vi "Update Any Values to UI.vi"(0 "Measurement Client Wrapper":refnum<class "Measurement Client Wrapper.lvclass">, 11 "error in":errorcluster) -> (4 "Measurement Client Wrapper out":refnum<class "Measurement Client Wrapper.lvclass">, 15 "error out":errorcluster)   [LabVIEW 2020, in "Measurement Client Wrapper.lvclass"]
uses:
  Measurement Client Wrapper.lvclass
  Measurement Client Wrapper.lvclass/Measurement Client Wrapper.ctl
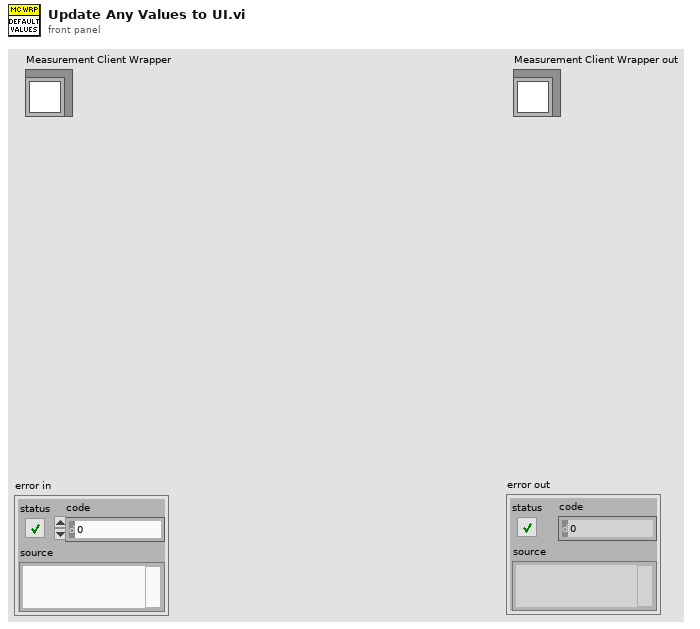
[diagram p1: front panel]
types:
  T1 = typedef "Measurement Client Wrapper.lvclass/MeasurementConfigurationParameters.ctl" = cluster{"protobuf_id":u32, "type":T2, "name":string, "repeated":bool}
  T2 = typedef "Measurement_client-release.lvlib/ni_measurements_v1_Type.ctl" = enum32{"TYPE_UNSPECIFIED", "TYPE_DOUBLE", "TYPE_FLOAT", "TYPE_INT64", "TYPE_UINT64", "TYPE_INT32", "TYPE_FIXED64", "TYPE_FIXED32", "TYPE_BOOL", "TYPE_STRING", "TYPE_GROUP", "TYPE_MESSAGE", "TYPE_BYTES", "TYPE_UINT32", "TYPE_ENUM", "TYPE_SFIXED32", "TYPE_SFIXED64", "TYPE_SINT32", "TYPE_SINT64"}
  T3 = typedef "Measurement Client Wrapper.lvclass/Control UI MetaData.ctl" = cluster{"Name":string, "Parent":string, "LabVIEW DataType":T4, "Measurement DataType":T2, "Value":variant, "1D Array?":bool}
  T4 = typedef "NI_Data Type.lvlib/Data Type.ctl" = enum8{"Invalid Type", "Void", "I8", "I16", "I32", "I64", "U8", "U16", "U32", "U64", "Single Float", "Double Float", "Extended Float", "Single Complex", "Double Complex", "Extended Complex", "Enum U8", "Enum U16", "Enum U32", "Enum U64", "Single Float With Unit", "Double Float With Unit", "Extended Float With Unit", "Single Complex with Unit", "Double Complex with Unit", "Extended Complex with Unit", "Boolean", "String", "Path", "Picture", "Tag", "Array", "Cluster", "Variant", "LV Variant", "Waveform", "Timestamp", "Digital Waveform", "Digital Data", "ExpressData", "Refnum", "External Data", "VI", "Poly VI", "LabVIEW Class Instance", "Fixed Point", "Set Collection", "Map Collection"}
  T5 = cluster{"type":T2, "repeated":bool, "Value":variant}
  T6 = cluster{"Measurement DataType":T2, "Array Dimension":bool, "Data":variant}[]
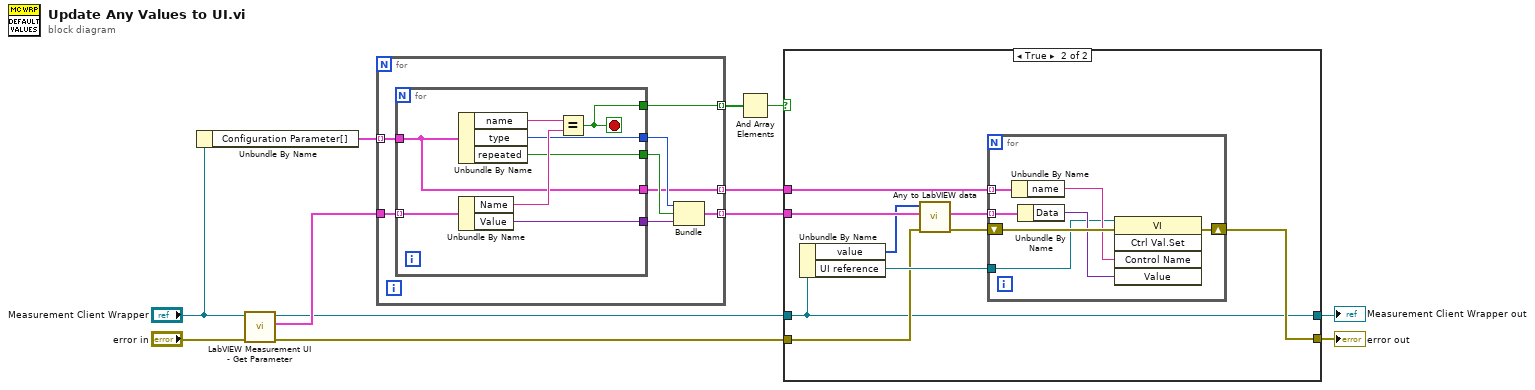
[diagram p0: block diagram]
diagram:
  n1 = Unbundle By Name("Measurement Client Wrapper") -> ("Configuration Parameter[]"=w9:T1[])
  n2 = call "LabVIEW Measurement UI - Get Parameter.vi"("error in"="error in", "Measurement Client Wrapper in"="Measurement Client Wrapper") -> ("error out"=w4:errorcluster, "UI Control Details[]"=w11:T3[], "Measurement Client Wrapper"=w5:refnum<class "Measurement Client Wrapper.lvclass">)  [unwired: 6 in, 1 out]
  n3 = for {
    tunnel: w9 -> [w19] mode=indexing
    tunnel: w11 -> [w20]
    tunnel: [w16] -> w3 mode=indexing
    tunnel: [w14] -> w7 mode=indexing
    tunnel: [w13] -> w6 mode=indexing
    n4 = for {
      tunnel: w20 -> [w28] mode=indexing
      tunnel: w19 -> [w22]
      tunnel: [w25] -> w17
      tunnel: [w24] -> w18
      tunnel: [w23] -> w15
      tunnel: [w22] -> w14
      tunnel: [w21] -> w13
      stop <- w21 stop-if-true
      n5 = Unbundle By Name(w22) -> ("name"=w26:string, "type"=w24:T2, "repeated"=w23:bool)
      n6 = Unbundle By Name(w28) -> ("Name"=w27:string, "Value"=w25:variant)
      n7 = Equal?(x=w26, y=w27) -> (x = y?=w21:bool)
    }
    n8 = Bundle("type"=w18, "repeated"=w15, "Value"=w17) -> (w16:T5)  [unwired: 1 in]
  }
  n9 = And Array Elements(Boolean array=w6) -> (logical AND=w2:bool)
  n10 = case shown="True" w2 {
    tunnel: [w30 w38] -> w10
    tunnel: w7 -> [_ w37]
    tunnel: w5 -> [w29 w32]
    tunnel: w4 -> [w30 w36]
    tunnel: w3 -> [_ w33]
    tunnel: [w29 w32] -> w1
    frame False {
    }
    frame True {
      n11 = Unbundle By Name(w32) -> ("value"=w31:u8[], "UI reference"=w39:refnum<vi>)
      n12 = call "Any to LabVIEW data.vi"("error in"=w36, "Data Order"=w33, "Buffer"=w31) -> ("error out"=w35:errorcluster, "Output Data"=w34:T6)  [unwired: 7 in]
      n13 = for {
        shift-right: [w45] -> w38
        shift-left: w35 -> [w46]
        tunnel: w37 -> [w43] mode=indexing
        tunnel: w34 -> [w42] mode=indexing
        tunnel: w39 -> [w40]
        n14 = Unbundle By Name(w43) -> ("name"=w44:string)
        n15 = Unbundle By Name(w42) -> ("Data"=w41:variant)
        n16 = invoke class="VI" method="Ctrl Val.Set"(reference=w40, error in=w46, "Control Name"=w44, "Value"=w41) -> (error out=w45:errorcluster)  [unwired: 1 in, 4 out]
      }
    }
  }
  "error out" <- w10
  "Measurement Client Wrapper out" <- w1
